vi "Datasheet Table Find Run to Use.vi"(10 "Run Data":T1[](array[typedef]), 11 "Run Select (Field=value)":string) -> (2 "Found Run?":bool, 3 "Run Information":T1)   [LabVIEW 2011]
uses:
  TDMS/TDMS Run.ctl
  TDMS/TDMS Channel (Sxx).ctl
  database/Fields/Field Record.ctl
  database/Fields/Field DataTypes.ctl
  database/Fields/Field NextItem.ctl
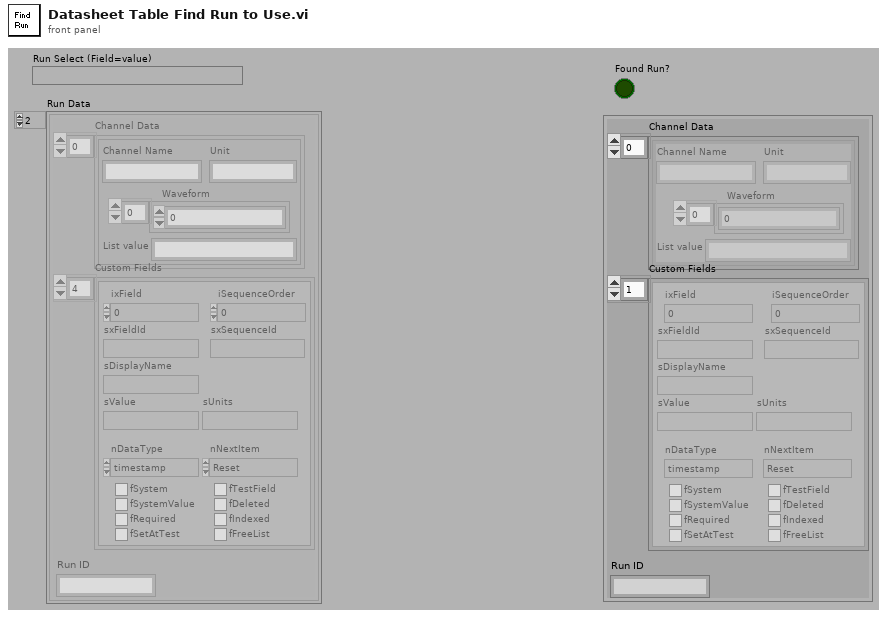
[diagram p1: front panel]
types:
  T1 = typedef "TDMS Run.ctl" = cluster{"Channel Data":T2[], "Custom Fields":T3[], "Run ID":string}
  T2 = typedef "TDMS Channel (Sxx).ctl" = cluster{"Channel Name":string, "Waveform":dbl[], "Unit":string, "List value":string}
  T3 = typedef "Field Record.ctl" = cluster{"ixField":i32, "iSequenceOrder":i32, "sxFieldId":string, "sxSequenceId":string, "sDisplayName":string, "sValue":string, "sUnits":string, "nDataType":T4, "nNextItem":T5, "fSystem":bool, "fSystemValue":bool, "fRequired":bool, "fSetAtTest":bool, "fTestField":bool, "fDeleted":bool, "fIndexed":bool, "fFreeList":bool}
  T4 = typedef "Field DataTypes.ctl" = enum32{"text", "numeric", "list", "timestamp", "boolean"}
  T5 = typedef "Field NextItem.ctl" = enum32{"Reset", "Retain", "Auto-Increment"}
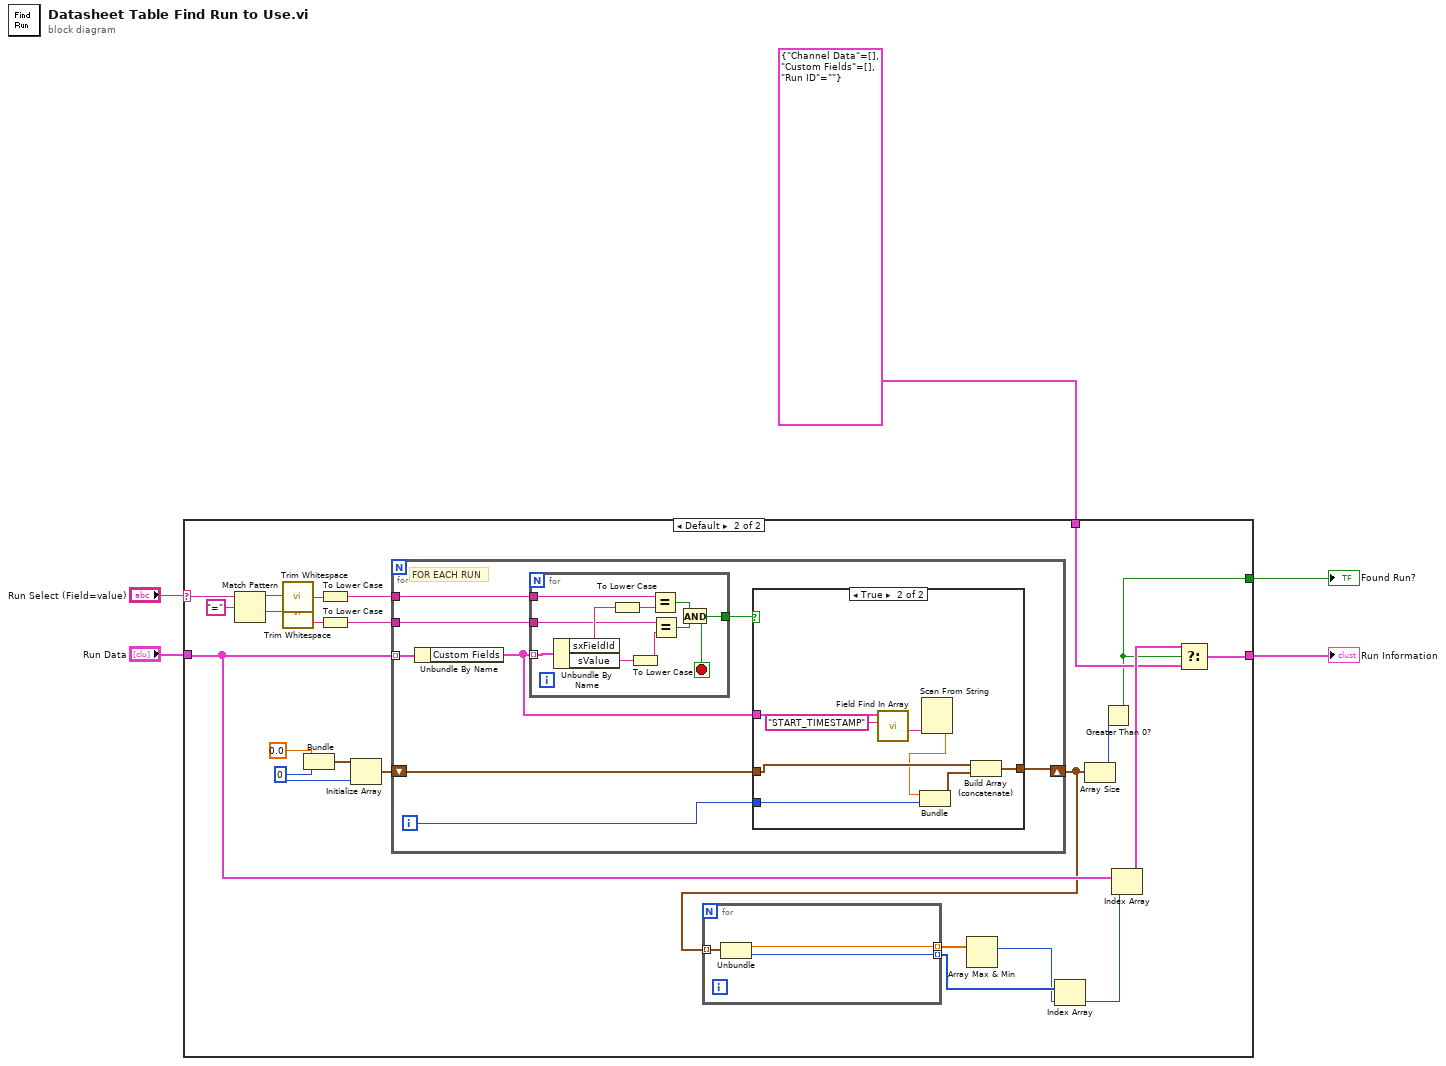
[diagram p0: block diagram]
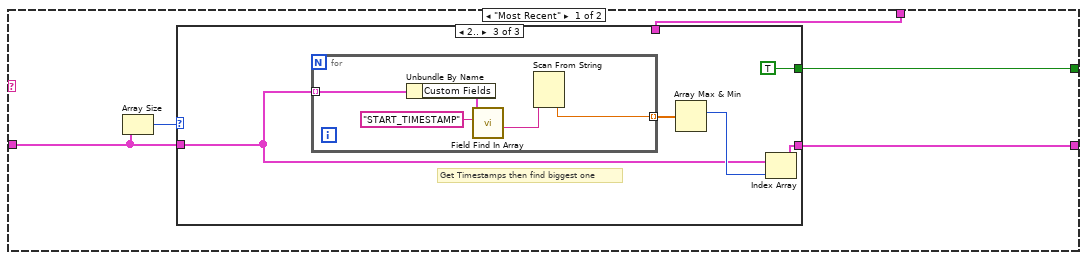
[diagram p2: hidden frame]
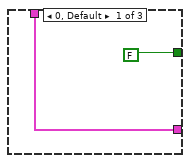
[diagram p3: hidden frame]
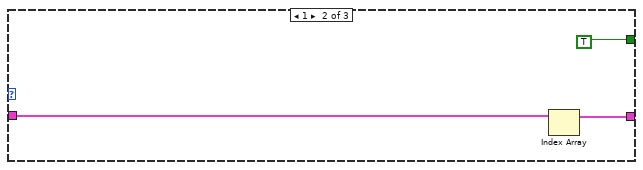
[diagram p4: hidden frame]
diagram:
  n1 = case shown="Default" "Run Select (Field=value)" {
    selector: "Run Select (Field=value)" -> [_ w48]
    tunnel: "Run Data" -> [w9 w41]
    tunnel: [w10 w38] -> w1
    tunnel: T1 {"Channel Data"=[], "Custom Fields"=[], "Run ID"=""} ("Run Information") -> [w6 w39]
    tunnel: [w7 w31] -> w2
    frame "Most Recent" {
      n2 = Array Size(array=w9) -> (size(s)=w8:i32)
      n3 = case shown="2.." w8 {
        tunnel: w9 -> [_ w14 w18]
        tunnel: [w11 w13 w17] -> w10
        tunnel: [FALSE TRUE TRUE] -> w7
        tunnel: w6 -> [w11 _ _]
        frame 0, Default {
        }
        frame 1 {
          n4 = Index Array(array=w14) -> (element=w13:T1)  [unwired: 1 in]
        }
        frame 2.. {
          # "Get Timestamps then find biggest one"
          n5 = for {
            tunnel: w18 -> [w25] mode=indexing
            tunnel: [w21] -> w20 mode=indexing
            n6 = Unbundle By Name(w25) -> ("Custom Fields"=w24:T3[])
            n7 = call "Field Find In Array.vi"("FieldID or Display Name(\"\")"="START_TIMESTAMP" ("FieldID or Display Name(\"\")"), "Field Array"=w24) -> ("sValue"=w22:string)  [unwired: 1 in, 8 out]
            n8 = Scan From String(input string=w22) -> (output 1=w21:dbl)  [unwired: 3 in, 4 out]
          }
          n9 = Array Max & Min(array=w20) -> (max index (indices)=w19:i32)  [unwired: 3 out]
          n10 = Index Array(array=w18, index=w19) -> (element=w17:T1)
        }
      }
    }
    frame Default {
      w33 = 0
      n11 = Match Pattern(string=w48, regular expression="=") -> (before substring=w46:string, after substring=w45:string)  [unwired: 3 out]
      n12 = call <vilib>:"Trim Whitespace.vi"("string"=w46) -> ("trimmed string"=w37:string)  [unwired: 1 in]
      n13 = call <vilib>:"Trim Whitespace.vi"("string"=w45) -> ("trimmed string"=w44:string)  [unwired: 1 in]
      n14 = Bundle(0.0, w33) -> (w35:cluster{dbl, i32})  [unwired: 1 out]
      n15 = To Lower Case(string=w37) -> (all lower case string=w43:string)
      n16 = To Lower Case(string=w44) -> (all lower case string=w42:string)
      n17 = Initialize Array(w35, w33) -> (w36:cluster{dbl, i32}[])
      n18 = for {
        tunnel: w41 -> [w59] mode=indexing
        tunnel: w43 -> [w58]
        tunnel: w42 -> [w57]
        shift-right: [w53] -> w30
        shift-left: w36 -> [w54]
        i -> [w52]
        # "FOR EACH RUN"
        n19 = Unbundle By Name(w59) -> ("Custom Fields"=w55:T3[])
        n20 = for {
          tunnel: w55 -> [w78] mode=indexing
          tunnel: w58 -> [w77]
          tunnel: w57 -> [w74]
          tunnel: [w69] -> w56
          stop <- w69 stop-if-true
          n21 = Unbundle By Name(w78) -> ("sxFieldId"=w76:string, "sValue"=w75:string)
          n22 = To Lower Case(string=w76) -> (all lower case string=w70:string)
          n23 = To Lower Case(string=w75) -> (all lower case string=w71:string)
          n24 = Equal?(x=w77, y=w70) -> (x = y?=w73:bool)
          n25 = Equal?(x=w74, y=w71) -> (x = y?=w72:bool)
          n26 = And(x=w73, y=w72) -> (x .and. y?=w69:bool)
        }
        n27 = case shown="True" w56 {
          tunnel: w55 -> [_ w66]
          tunnel: w54 -> [w60 w64]
          tunnel: [w60 w65] -> w53
          tunnel: w52 -> [_ w61]
          frame False {
          }
          frame True {
            n28 = call "Field Find In Array.vi"("FieldID or Display Name(\"\")"="START_TIMESTAMP" ("FieldID or Display Name(\"\")"), "Field Array"=w66) -> ("sValue"=w67:string)  [unwired: 1 in, 8 out]
            n29 = Scan From String(input string=w67) -> (output 1=w62:dbl)  [unwired: 3 in, 4 out]
            n30 = Bundle(w62, w61) -> (w63:cluster{dbl, i32})  [unwired: 1 out]
            n31 = Build Array (concatenate)(w64, w63) -> (w65:cluster{dbl, i32}[])
          }
        }
      }
      n32 = for {
        tunnel: w30 -> [w51] mode=indexing
        tunnel: [w50] -> w29 mode=indexing
        tunnel: [w49] -> w28 mode=indexing
        n33 = Unbundle(w51) -> (w50:dbl, w49:i32)
      }
      n34 = Array Max & Min(array=w29) -> (max index (indices)=w27:i32)  [unwired: 3 out]
      n35 = Index Array(array=w28, index=w27) -> (element=w26:i32)
      n36 = Array Size(array=w30) -> (size(s)=w32:i32)
      n37 = Greater Than 0?(x=w32) -> (x > 0?=w31:bool)
      n38 = Index Array(array=w41, index=w26) -> (element=w40:T1)
      n39 = Select(t=w40, s=w31, f=w39) -> (s? t:f=w38:T1)
    }
  }
  "Run Information" <- w1
  "Found Run?" <- w2
